vi "Remove Number From Array.vi"(1 "Number":dbl format="%#_13g", 2 "Input array":dbl[](array[numeric])) -> (0 "output array":dbl[](array[numeric]))   [LabVIEW 2020]
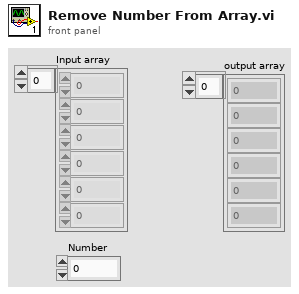
[diagram p1: front panel]
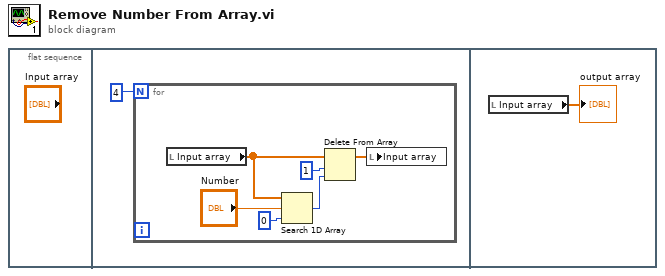
[diagram p0: block diagram]
diagram:
  n1 = flat-sequence {
    frame #0 {
    }
    frame #1 {
      n2 = for {
        N: 4 -> [_]
        n3 = local read "Input array"() -> (w3:dbl[])
        n4 = Search 1D Array(1D array=w3, element="Number", start index (0)=0) -> (index of element=w4:i32)
        n5 = Delete From Array(array=w3, length=1, index=w4) -> (array with subset deleted=w2:dbl[])  [unwired: 1 out]
        n6 = local write "Input array"(w2) -> ()
      }
    }
    frame #2 {
      n7 = local read "Input array"() -> (→"output array":dbl[])
    }
  }
